vi "SLL DE Split Virtual Channels.vi"(7 "GlobalChans":refnum<k21>[](array[refnum]), 8 "error in (no error)":errorcluster, 11 "All Device Names (Chassis & Module)":cluster{"New element":tag[]}[](array[cluster])) -> (0 "error out":errorcluster, 2 "Channel Array":cluster{"Device Channel List":string[]}[](array[cluster]), 3 "Error?":bool)   [LabVIEW 2013]
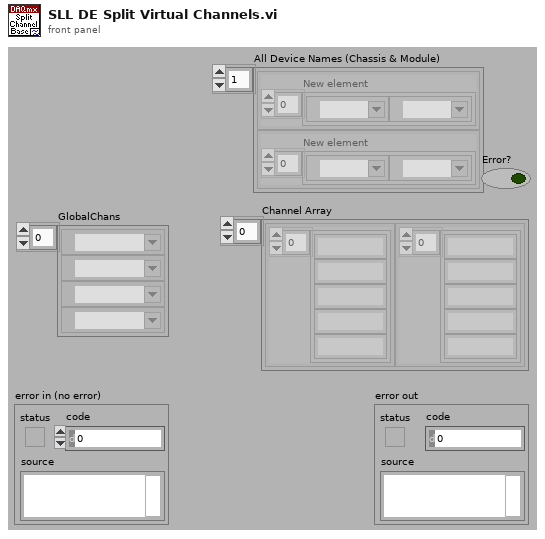
[diagram p1: front panel]
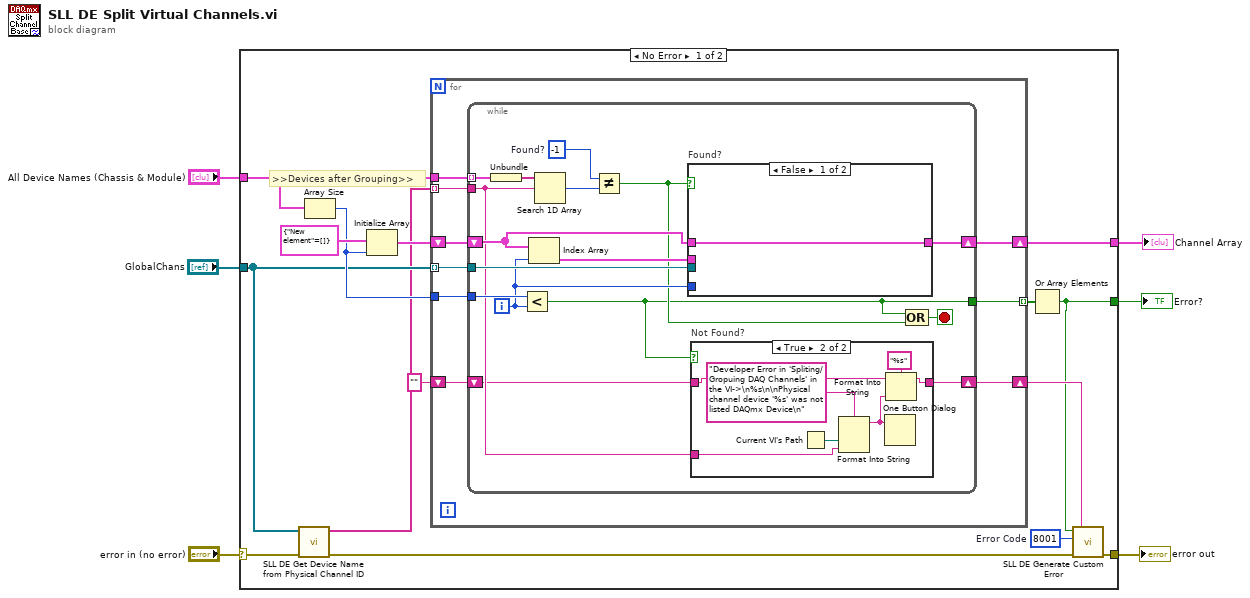
[diagram p0: block diagram]
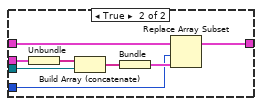
[diagram p3: hidden frame]
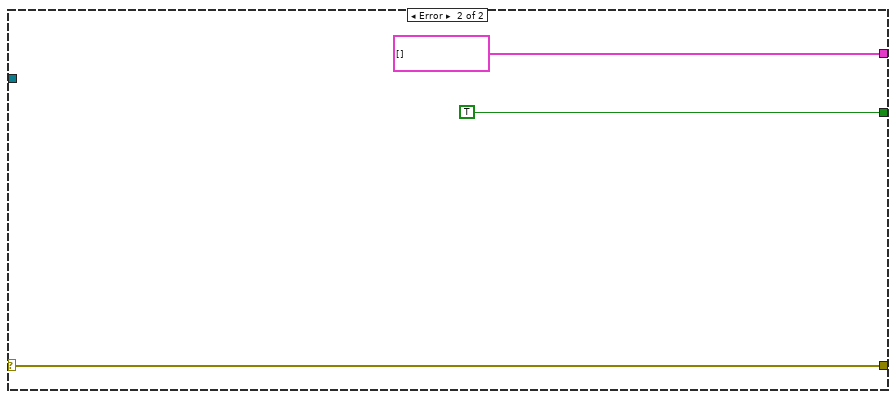
[diagram p4: hidden frame]
diagram:
  n1 = case shown="No Error" "error in (no error)" {
    selector: "error in (no error)" -> [w16 w66]
    tunnel: [w7 cluster{"New element":string[]}[] []] -> w6
    tunnel: "GlobalChans" -> [w15 _]
    tunnel: "All Device Names (Chassis & Module)" -> [w17 _]
    tunnel: [w9 TRUE] -> w3
    tunnel: [w11 w66] -> w1
    frame No Error {
      w8 = 8001  # Error Code
      # ">>Devices after Grouping>>"
      n2 = call "SLL DE Get Device Name from Physical Channel ID.vi"("error in (no error)"=w16, "GlobalChans"=w15) -> ("error out"=w12:errorcluster, "Dev Names from Physical Channel"=w14:tag[])  [unwired: 8 in]
      n3 = Array Size(array=w17) -> (size(s)=w20:i32)
      n4 = Initialize Array(cluster{"New element":string[]} {"New element"=[]}, w20) -> (w19:cluster{"New element":string[]}[])
      n5 = for {
        tunnel: w15 -> [w26] mode=indexing
        tunnel: w17 -> [w30]
        tunnel: w20 -> [w29]
        shift-right: [w27] -> w7
        shift-left: w19 -> [w28]
        tunnel: [w24] -> w18 mode=indexing
        tunnel: w14 -> [w25] mode=indexing
        shift-right: [w23] -> w10
        shift-left: "" -> [w22]
        n6 = while {
          tunnel: w30 -> [w46] mode=indexing
          tunnel: w25 -> [w33]
          tunnel: w29 -> [w43]
          shift-right: [w39] -> w27
          shift-left: w28 -> [w40]
          tunnel: w26 -> [w41]
          tunnel: [w34] -> w24
          shift-right: [w32] -> w23
          shift-left: w22 -> [w31]
          i -> [w38]
          stop <- w44 stop-if-true
          w36 = -1  # Found?
          n7 = Unbundle(w46) -> ("New element"=w45:tag[])
          n8 = Less?(x=w43, y=w38) -> (x < y?=w34:bool)
          n9 = Index Array(array=w40, index=w38) -> (element=w42:cluster{"New element":string[]})
          n10 = Search 1D Array(1D array=w45, element=w33) -> (index of element=w37:i32)  [unwired: 1 in]
          n11 = Not Equal?(x=w36, y=w37) -> (x != y?=w35:bool)
          n12 = case "Found?" shown="False" w35 {
            tunnel: w42 -> [_ w63]
            tunnel: w41 -> [_ w61]
            tunnel: w40 -> [w55 w58]
            tunnel: [w55 w57] -> w39
            tunnel: w38 -> [_ w56]
            frame False {
            }
            frame True {
              n13 = Unbundle(w63) -> ("New element"=w62:string[])
              n14 = Build Array (concatenate)(w62, w61) -> (w60:string[])
              n15 = Bundle(w60) -> (w59:cluster{string[]})  [unwired: 1 in]
              n16 = Replace Array Subset(array=w58, new element=w59, index=w56) -> (w57:cluster{"New element":string[]}[])
            }
          }
          n17 = case "Not Found?" shown="True" w34 {
            tunnel: w33 -> [_ w52]
            tunnel: [w47 w48] -> w32
            tunnel: w31 -> [w47 w51]
            frame False {
            }
            frame True {
              n18 = Current VI's Path() -> (path=w53:path)
              n19 = Format Into String(format string="Developer Error in 'Spliting/Gropuing DAQ Channels' in the VI->\n%s\n\nPhysical channel device '%s' was not listed DAQmx Device\n" ("message"), w53, w52) -> (resulting string=w49:string)  [unwired: 2 in, 1 out]
              n20 = One Button Dialog(message=w49) -> ()  [unwired: 1 in, 1 out]
              n21 = Format Into String(format string="%s", initial string=w51, w49) -> (resulting string=w48:string)  [unwired: 1 in, 1 out]
            }
          }
          n22 = Compound Arithmetic op=OR(w34, w35) -> (w44:bool)
        }
      }
      n23 = Or Array Elements(Boolean array=w18) -> (logical OR=w9:bool)
      n24 = call "SLL DE Generate Custom Error.vi"("Case Name"=w10, "error in"=w12, "Error Code (0)"=w8, "Error? (T)"=w9) -> ("error out"=w11:errorcluster)  [unwired: 7 in]
    }
    frame Error {
    }
  }
  "error out" <- w1
  "Channel Array" <- w6
  "Error?" <- w3
